vi "Read Sequential Address.vi"(5 "BCI-1553-RSP":refnum<k21>, 6 "Target ID":u8, 7 "BCI-1553 Device":refnum<k21>, 9 "Count":u16, 10 "Address":u16) -> ()   [LabVIEW 2020, in "BCI-1553 RT Interface.lvlib"]
doc: "Performs sequential address reading."
uses:
  BCI-1553 RT Interface.lvlib
  <vilib>/rvi/Emulation/niFpgaGetClockAttributes.vi
  <vilib>/rvi/Emulation/niFpgaSctlEmulationGetInTimedLoop.vi
  <vilib>/rvi/Emulation/niFpgaEmulationReportErrorSimple.vi
  <vilib>/rvi/eio/common/nirviEmuTemplateMethod_errors.vi
  <vilib>/rvi/DataTransferAndStorage/Container/Common/niFpgaContainerExecOnDevCompGetState.vi
  <vilib>/rvi/Emulation/niFpgaEmulationIsFPGAContextNoSignature.vi
  <vilib>/rvi/errors/niFpgaSetErrorForExecOnDevCompSimple.vi
  <vilib>/rvi/eio/common/nirviEmuReportErrorAndStop.vi
  <vilib>/rvi/DataTransferAndStorage/Container/Common/niFpgaContainerGetUniqueNameForEmu.vi
  <vilib>/rvi/FIFO/Fifo_Resource/nirvififoEmulationSetSize.vi
  <vilib>/rvi/FIFO/Fifo_Resource/nirviFifoEmulationQueueMgr.vi
  <instcachedir>/0/nirviFifoEmulationQueueMgr_E5CAEC123FF24DC58D834DCA3CDAA9B5.lvgen/nirviFifoEmulationQueueMgr_E5CAEC123FF24DC58D834DCA3CDAA9B5_001.vi
  <vilib>/rvi/FIFO/Fifo_Resource/nirvififoEmulationDetermineInputValidOut.vi
  <vilib>/rvi/FIFO/Fifo_Resource/nirvififoEmulationCreateLock.vi
  <vilib>/rvi/Emulation/niFpgaProcessEmulError.vi
  <vilib>/rvi/FIFO/Fifo_Resource/nirvififoEmulationObtainLock.vi
  <vilib>/rvi/FIFO/Fifo_Resource/nirvififoEmulationReleaseLock.vi
  <vilib>/rvi/occurrence/nirviWaitOnOccurrenceBase.vi
  <vilib>/rvi/errors/nirviReportUnexpectedCaseInternalError.vi
  <vilib>/rvi/errors/nirviReportUnexpectedCaseInternalError (U32).vi
  <vilib>/Utility/error.llb/Clear Errors.vi
  <vilib>/rvi/interface/RandomDataEmulation/niFpgaRandomDataHandleErrors.vi
  <vilib>/rvi/Emulation/niFpgaCriticalErrorInLSC.vi
  <vilib>/eio/EIOMethodNode/EIOMethodNode.xnode
  <vilib>/rvi/DataTransferAndStorage/Container/XNode/niFpgaContainer.xnode
  <vilib>/rvi/FIFO/Fifo_Resource/niFpgaFifoEmulationRefIn.vi
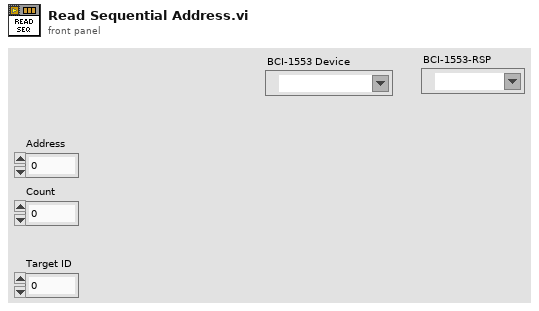
[diagram p1: front panel]
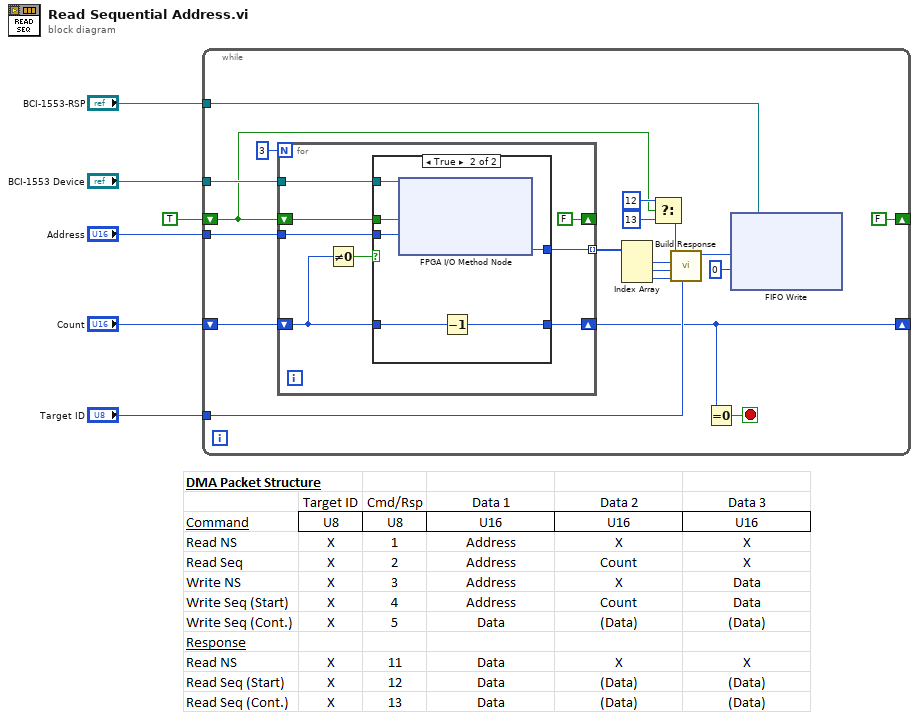
[diagram p0: block diagram]
diagram:
  n1 = while {
    shift-right: [FALSE] -> _
    shift-left: TRUE -> [w13]
    tunnel: "BCI-1553 Device" -> [w22]
    tunnel: "Address" -> [w21]
    shift-right: [w7] -> _
    shift-left: "Count" -> [w23]
    tunnel: "Target ID" -> [w8]
    tunnel: "BCI-1553-RSP" -> [w12]
    stop <- w9 stop-if-true
    n2 = for {
      N: 3 -> [_]
      tunnel: w22 -> [w33]
      shift-right: [FALSE] -> _
      shift-left: w13 -> [w32]
      tunnel: w21 -> [w31]
      shift-right: [w27] -> w7
      shift-left: w23 -> [w28]
      tunnel: [w26] -> w20 mode=indexing
      n3 = Not Equal To 0?(x=w28) -> (x != 0?=w29:bool)
      n4 = case shown="True" w29 {
        tunnel: w33 -> [_ w40]
        tunnel: w32 -> [_ w39]
        tunnel: w31 -> [_ w38]
        tunnel: w28 -> [w34 w37]
        tunnel: [w34 w36] -> w27
        tunnel: [_ w35] -> w26
        frame False {
        }
        frame True {
          n5 = xnode "FPGA I/O Method Node"("FPGA I/O In"=w40, "Initialize"=w39, "Address"=w38) -> ("Data"=w35:u16)  [unwired: 1 out]
          n6 = Decrement(x=w37) -> (x-1=w36:u16)
        }
      }
    }
    n7 = Index Array(array=w20) -> (element #1=w19:u16, element #2=w18:u16, element #3=w17:u16)  [unwired: 3 in]
    n8 = Select(t=u8 12 ("Response"), s=w13, f=u8 13 ("Response")) -> (s? t:f=w14:u8)
    n9 = call "Build Response.vi"("Target ID"=w8, "Data 3"=w17, "Data 2"=w18, "Data 1"=w19, "Response"=w14) -> ("Response Value"=w11:u64)  [unwired: 6 in]
    n10 = Equal To 0?(x=w7) -> (x = 0?=w9:bool)
    n11 = xnode "FIFO Write"("Element"=w11, "Timeout"=0, "FIFO In"=w12) -> ()  [unwired: 2 out]
  }
